vi "Read Step requesting configuration.vi"(8 "error in (no error)":errorcluster, 11 "HW Configuration in":refnum<class "HW Configuration.lvclass">) -> (0 "error out":errorcluster, 2 "Step requesting configuration":string, 3 "HW Configuration out":refnum<class "HW Configuration.lvclass">)   [LabVIEW 2017, in "Hardware.lvlib" / "HW Configuration.lvclass"]
uses:
  HW Configuration.lvclass
  HW Configuration.lvclass/HW Configuration.ctl
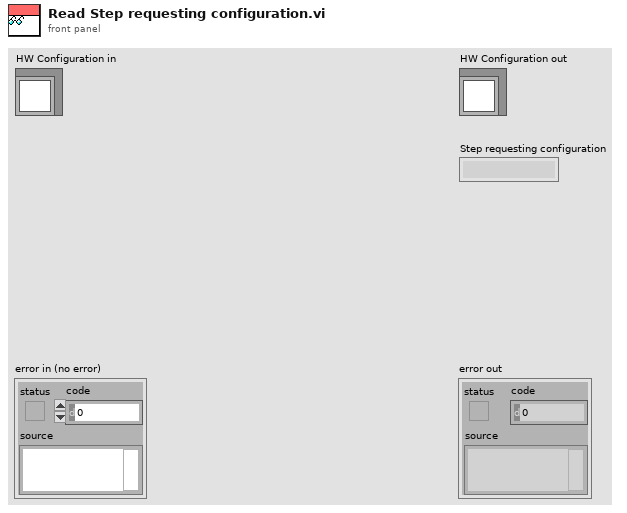
[diagram p1: front panel]
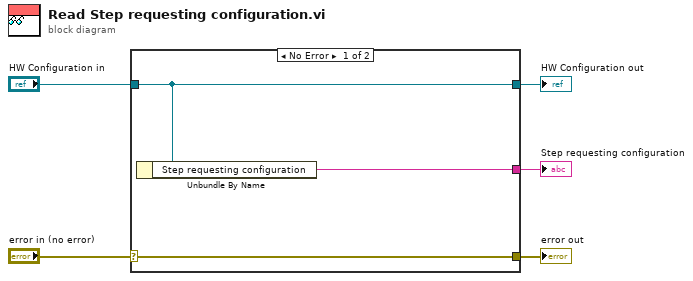
[diagram p0: block diagram]
diagram:
  n1 = case shown="No Error" "error in (no error)" {
    selector: "error in (no error)" -> [w8 w9]
    tunnel: [w8 w9] -> w4
    tunnel: [w7 w10] -> w2
    tunnel: "HW Configuration in" -> [w7 w10]
    tunnel: [w6 _] -> w1
    frame No Error {
      n2 = Unbundle By Name(w7) -> ("Step requesting configuration"=w6:string)
    }
    frame Error {
    }
  }
  "error out" <- w4
  "HW Configuration out" <- w2
  "Step requesting configuration" <- w1
